vi "GlobalGyro.vi"() -> ()   [LabVIEW 2015]
panel:
  out "DesiredGyroValue":dbl
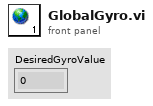
[diagram p1: front panel]
diagram:
